vi "SQL查询.vi"(7 "condition":string, 9 "columns":string[](array[string]), 10 "table输入":string(combo), 11 "database":string(combo)) -> (0 "error out":errorcluster, 2 "columns输出":string[](array[string]), 3 "data":string[][](table))   [LabVIEW 2016, in "数据传输系统.lvlib"]
uses:
  <vilib>/Utility/sysdir.llb/System Directory Type.ctl
  <vilib>/addons/database/Connection.llb/DB Tools Open Connec (String).vi
  <vilib>/addons/database/_DB Variant To Data/Database Variant To Data.xnode
  <vilib>/addons/database/NI_Database_API.lvlib
panel:
  out "子数组":string[](array[string])
  in  "error in (no error)":errorcluster
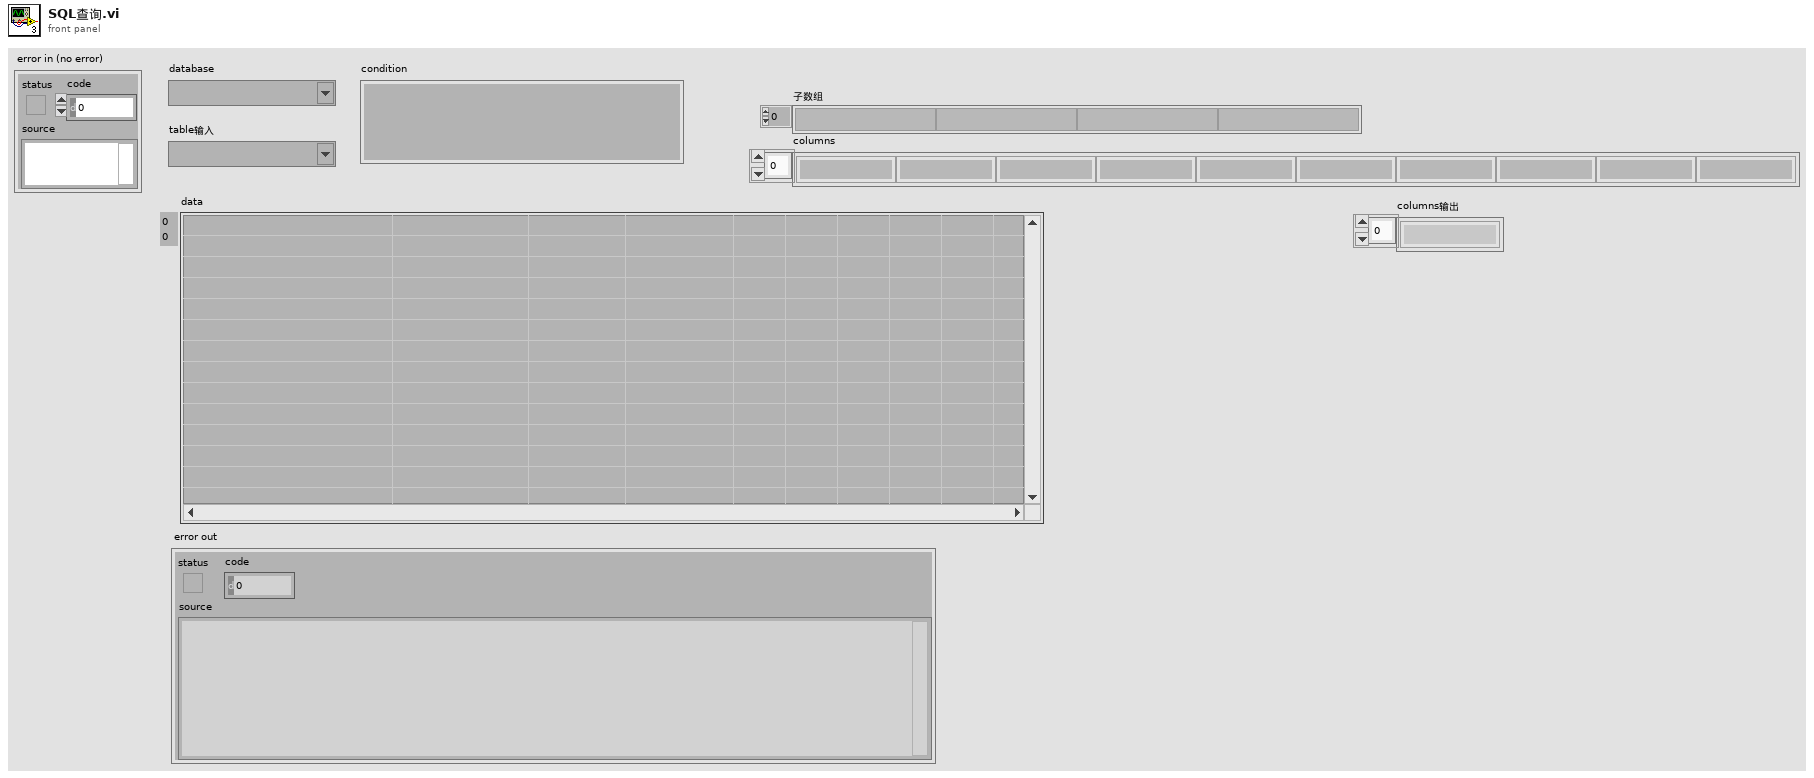
[diagram p1: front panel]
types:
  T1 = typedef "System Directory Type.ctl" = i32
  T2 = typedef "NI_Database_API.lvlib/Conn ObjectReference.ctl" = refnum<k1>
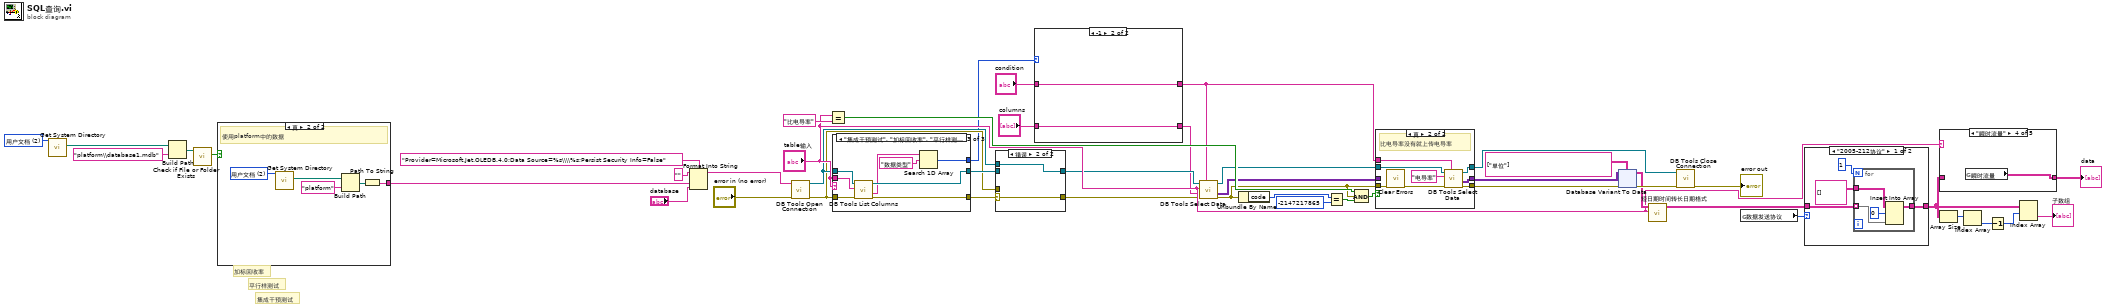
[diagram p0: block diagram]
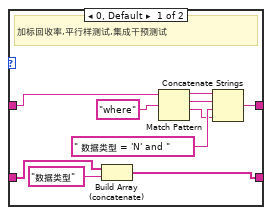
[diagram p2: hidden frame]
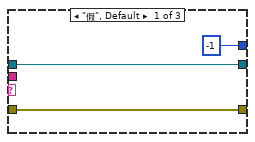
[diagram p4: hidden frame]
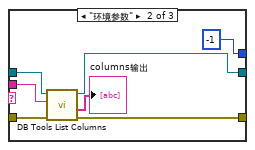
[diagram p5: hidden frame]
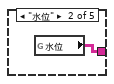
[diagram p8: hidden frame]
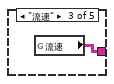
[diagram p9: hidden frame]
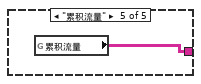
[diagram p10: hidden frame]
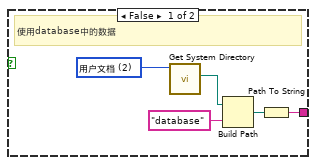
[diagram p11: hidden frame]
diagram:
  w31 = T1 2 items=["用户目录"=0, "用户桌面"=1, "用户文档"=2, "用户应用程序数据"=3, "用户设置"=4, "用户临时目录"=5, "公共文档"=6, "公共应用程序数据"=7, "公共设置"=8, "公共缓存"=13, "系统核心库"=9, "系统安装库"=10, "应用程序文件"=11, "启动盘根目录"=12] ("system directory type")
  # "集成干预测试"
  # "平行样测试"
  # "加标回收率"
  n1 = call <vilib>:"Get System Directory.vi"("system directory type"=w31) -> ("system directory"=w32:path)  [unwired: 10 in]
  n2 = Build Path(base path=w32, name or relative path="platform\\database1.mdb" ("condition")) -> (appended path=w30:path)
  n3 = call <vilib>:"Check if File or Folder Exists.vi"("path"=w30) -> ("file or folder exists?"=w28:bool)  [unwired: 8 in, 2 out]
  n4 = case shown="真" w28 {
    tunnel: [w48 w53] -> w27
    frame False {
      w51 = T1 2 items=["用户目录"=0, "用户桌面"=1, "用户文档"=2, "用户应用程序数据"=3, "用户设置"=4, "用户临时目录"=5, "公共文档"=6, "公共应用程序数据"=7, "公共设置"=8, "公共缓存"=13, "系统核心库"=9, "系统安装库"=10, "应用程序文件"=11, "启动盘根目录"=12] ("system directory type")
      # "使用database中的数据"
      n5 = call <vilib>:"Get System Directory.vi"("system directory type"=w51) -> ("system directory"=w50:path)  [unwired: 10 in]
      n6 = Build Path(base path=w50, name or relative path="database" ("condition")) -> (appended path=w52:path)
      n7 = Path To String(path=w52) -> (string=w48:string)
    }
    frame True {
      w57 = T1 2 items=["用户目录"=0, "用户桌面"=1, "用户文档"=2, "用户应用程序数据"=3, "用户设置"=4, "用户临时目录"=5, "公共文档"=6, "公共应用程序数据"=7, "公共设置"=8, "公共缓存"=13, "系统核心库"=9, "系统安装库"=10, "应用程序文件"=11, "启动盘根目录"=12] ("system directory type")
      # "使用platform中的数据"
      n8 = call <vilib>:"Get System Directory.vi"("system directory type"=w57) -> ("system directory"=w56:path)  [unwired: 10 in]
      n9 = Build Path(base path=w56, name or relative path="platform" ("condition")) -> (appended path=w54:path)
      n10 = Path To String(path=w54) -> (string=w53:string)
    }
  }
  n11 = Format Into String(format string="Provider=Microsoft.Jet.OLEDB.4.0;Data Source=%s\\\\%s;Persist Security Info=False" ("格式字符串"), initial string="" ("初始字符串"), w27, "database") -> (resulting string=w40:string)  [unwired: 1 in, 1 out]
  n12 = call-poly <vilib>:"DB Tools Open Connection.vi"("error in (no error)"="error in (no error)", "connection information"=w40) -> ("error out"=w6:errorcluster, "connection reference"=w8:T2)  [unwired: 6 in]
  n13 = Equal?(x="table输入", y="比电导率") -> (x = y?=w24:bool)
  n14 = case shown="\"集成干预测试\", \"加标回收率\", \"平行样测试\"" "table输入" {
    tunnel: w8 -> [w60 w67 w75]
    tunnel: w6 -> [w59 w66 w73]
    tunnel: [w60 w65 w72] -> w10
    tunnel: [w59 w64 w71] -> w11
    tunnel: "table输入" -> [_ w63 w74]
    tunnel: [-1 ("index of element") -1 ("index of element") w68] -> w5
    frame "假", Default {
    }
    frame "环境参数" {
      n15 = call <vilib>:"DB Tools List Columns.vi"("error in (no error)"=w66, "table"=w63, "connection reference"=w67) -> ("error out"=w64:errorcluster, "columns"=→"columns输出":string[], "connection reference out"=w65:T2)  [unwired: 1 in, 1 out]
    }
    frame "集成干预测试", "加标回收率", "平行样测试" {
      n16 = call <vilib>:"DB Tools List Columns.vi"("error in (no error)"=w73, "table"=w74, "connection reference"=w75) -> ("error out"=w71:errorcluster, "columns"=w70:string[], "connection reference out"=w72:T2)  [unwired: 1 in, 1 out]
      n17 = Search 1D Array(1D array=w70, element="数据类型" ("元素")) -> (index of element=w68:i32)  [unwired: 1 in]
    }
  }
  n18 = case shown="错误" w11 {
    selector: w11 -> [_ w78]
    tunnel: w10 -> [w77 _]
    tunnel: [w77 w79] -> w9
    tunnel: w8 -> [_ w79]
    tunnel: [w76 w78] -> w7
    tunnel: w6 -> [w76 _]
    frame No Error {
    }
    frame Error {
    }
  }
  n19 = case "条件结构" shown="-1" w5 {
    tunnel: "condition" -> [w87 w90]
    tunnel: "columns" -> [w89 w91]
    tunnel: [w81 w91] -> w2
    tunnel: [w80 w90] -> w1
    frame 0, Default {
      # "加标回收率,平行样测试,集成干预测试"
      n20 = Build Array (concatenate)(w89, "数据类型" ("元素")) -> (w81:string[])
      n21 = Match Pattern(string=w87, regular expression="where" ("正则表达式")) -> (before substring=w85:string, match substring=w84:string, after substring=w82:string)  [unwired: 1 in, 1 out]
      n22 = Concatenate Strings(w85, w84, " 数据类型 = 'N' and " ("字符串"), w82) -> (w80:string)
    }
    frame -1 {
    }
  }
  n23 = call <vilib>:"DB Tools Select Data.vi"("condition"=w1, "error in (no error)"=w7, "columns"=w2, "table"="table输入", "connection reference"=w9) -> ("error out"=w17:errorcluster, "data"=w19:variant[][], "connection reference out"=w22:T2)  [unwired: 1 in]
  n24 = Unbundle By Name(w17) -> ("code"=w16:i32)
  n25 = Equal?(x=w16, y=-2147217865 ("code")) -> (x = y?=w14:bool)
  n26 = Compound Arithmetic op=AND ("复合运算")(w24, w17, w14) -> (w23:bool)
  n27 = case shown="真" w23 {
    tunnel: w1 -> [_ w102]
    tunnel: w22 -> [w94 w101]
    tunnel: [w94 w96] -> w21
    tunnel: [w93 w97] -> w20
    tunnel: w19 -> [w93 _]
    tunnel: w17 -> [w92 w99]
    tunnel: [w92 w95] -> w18
    frame False {
    }
    frame True {
      # "比电导率没有就上传电导率"
      n28 = call <vilib>:"Clear Errors.vi"("error in (no error)"=w99) -> ("error out"=w98:errorcluster)  [unwired: 5 in, 1 out]
      n29 = call <vilib>:"DB Tools Select Data.vi"("condition"=w102, "error in (no error)"=w98, "table"="电导率", "connection reference"=w101) -> ("error out"=w95:errorcluster, "data"=w97:variant[][], "connection reference out"=w96:T2)  [unwired: 2 in]
    }
  }
  n30 = xnode "Database Variant To Data"("database variant"=w20, "error in (no error)"=w18, "type"=string[][] [["单位"]]) -> ("data"=w39:string[][], "error out"=w44:errorcluster)
  n31 = call "短日期时间转长日期格式.vi"("table输入"="table输入", "data"=w39) -> ("输出数组"=w38:string[][])  [unwired: 9 in]
  n32 = call <vilib>:"DB Tools Close Connection.vi"("error in (no error)"=w44, "connection reference"=w21) -> ("error out"=→"error out":errorcluster)  [unwired: 5 in]
  n33 = global read "断电保存全局.vi" "数据发送协议"() -> (w37:enum16{"2005-212协议", "2017-212协议"})
  n34 = case shown="\"2005-212协议\"" w37 {
    tunnel: w38 -> [w104 w111]
    tunnel: [w103 w111] -> w26
    frame "2005-212协议" {
      n35 = for {
        N: 1 -> [_]
        tunnel: string[][] [] ("data") -> [w110]
        tunnel: w104 -> [w109] mode=indexing
        tunnel: [w107] -> w103
        n36 = Insert Into Array(array=w110, index (row)=0 ("索引 (行)"), new element=w109) -> (w107:string[][])  [unwired: 1 in]
      }
    }
    frame "2017-212协议", Default {
    }
  }
  n37 = case shown="\"瞬时流量\"" "table输入" {
    tunnel: w26 -> [w112 _ _ _ _]
    tunnel: [w112 w113 w114 w115 w116] -> w13
    frame Default {
    }
    frame "水位" {
      n38 = global read "全局流量数据小时.vi" "水位"() -> (w113:string[][])
    }
    frame "流速" {
      n39 = global read "全局流量数据小时.vi" "流速"() -> (w114:string[][])
    }
    frame "瞬时流量" {
      n40 = global read "全局流量数据小时.vi" "瞬时流量"() -> (w115:string[][])
    }
    frame "累积流量" {
      n41 = global read "全局流量数据小时.vi" "累积流量"() -> (w116:string[][])
    }
  }
  "data" <- w13
  n42 = Array Size(array=w26) -> (size(s)=w36:i32[])
  n43 = Index Array(array=w36) -> (element=w34:i32)  [unwired: 1 in]
  n44 = Decrement(x=w34) -> (x-1=w33:i32)
  n45 = Index Array(array=w26, index (row)=w33) -> (element=→"子数组":string[])  [unwired: 1 in]
